vi "Read_AVI_to_Array.vi"(8 "Error in (no error)":errorcluster, 11 "AVI Path":path) -> (0 "Error out":errorcluster, 2 "Data Array":string[](array[string]), 3 "Image Array":T1[](array[plugin-control]))   [LabVIEW 2012]
doc: "This example shows how to read and write both image information and data to an AVI file. The example also shows how to read a specific frame in an AVI file. The VI opens an existing AVI file, adds time stamp information, sample waveform data, and writes a sample image and the data to a new AVI file. You then can read the image and data associated with a specific frame. Use the Flatten To String and Unflatten From String functions to write and read data in AVI files."
uses:
  <vilib>/vision/Image Controls.llb/IMAQ Image.ctl
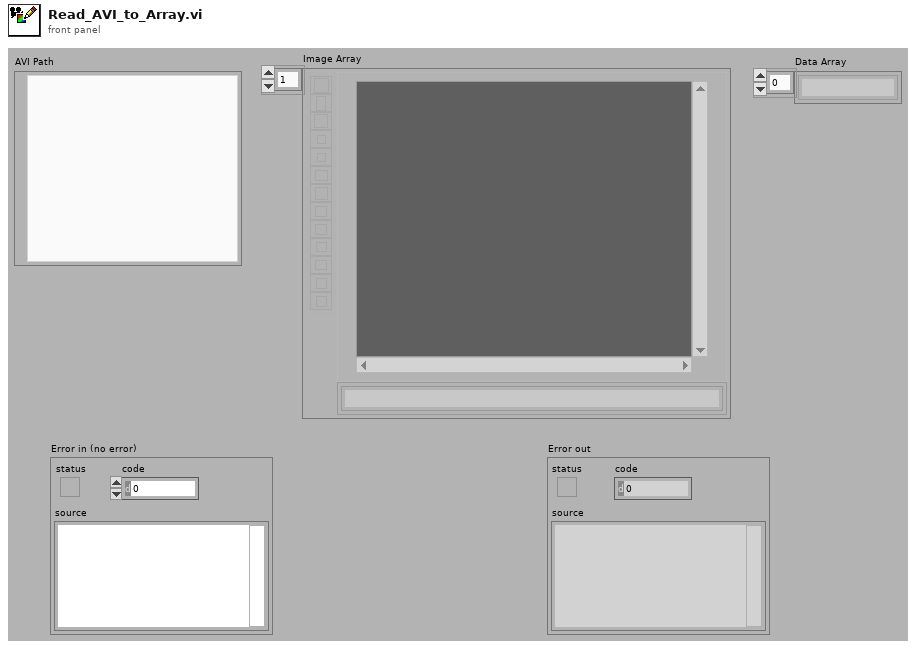
[diagram p1: front panel]
types:
  T1 = typedef "IMAQ Image.ctl" = refnum<image>
  T2 = typedef "Image Type" = u32
  T3 = typedef "AviRefnum.ctl" = refnum<k1>
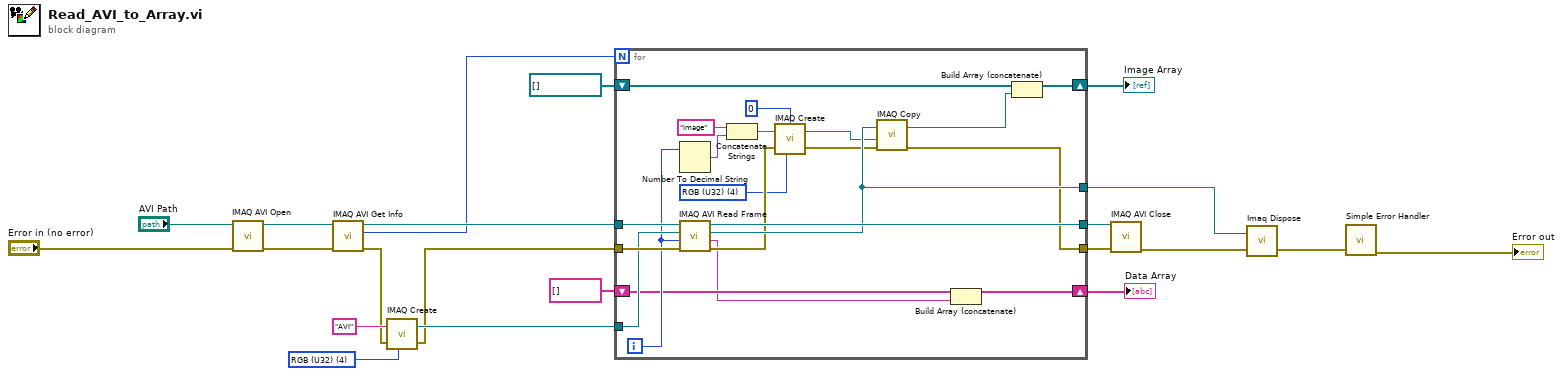
[diagram p0: block diagram]
diagram:
  w10 = T2 4 items=["Grayscale (U8)", "Grayscale (I16)", "Grayscale (SGL)", "Complex (CSG)", "RGB (U32)", "HSL (U32)", "RGB (U64)", "Grayscale (U16)"] ("Image Type")
  n1 = call "IMAQ AVI Open"("error in (no error)"="Error in (no error)", "AVI Path"="AVI Path") -> ("error out"=w14:errorcluster, "Avi Refnum"=w13:T3)  [unwired: 8 out]
  n2 = call "IMAQ AVI Get Info"("error in (no error)"=w14, "Avi Refnum"=w13) -> ("error out"=w8:errorcluster, "Number of Frames"=w9:u32, "Avi Refnum (duplicate)"=w12:T3)  [unwired: 5 in, 2 out]
  n3 = call "IMAQ Create"("Image Name"="AVI", "Image Type"=w10, "error in (no error)"=w8) -> ("New Image"=w19:T1, "error out"=w6:errorcluster)  [unwired: 1 in, 1 out]
  n4 = for {
    N: w9 -> [_]
    tunnel: [w38] -> w17
    tunnel: w19 -> [w39]
    tunnel: [w22] -> w16
    tunnel: [w40] -> w18
    tunnel: w12 -> [w42]
    tunnel: w6 -> [w41]
    shift-right: [w36] -> w1
    shift-left: T1[] [] ("Image Array") -> [w37]
    shift-right: [w25] -> w2
    shift-left: string[] [] ("Data Array") -> [w26]
    i -> [w27]
    w28 = T2 4 items=["Grayscale (U8)", "Grayscale (I16)", "Grayscale (SGL)", "Complex (CSG)", "RGB (U32)", "HSL (U32)", "RGB (U64)", "Grayscale (U16)"] ("Image Type")
    n5 = Number To Decimal String(number=w27) -> (decimal integer string=w33:string)  [unwired: 1 in]
    n6 = call "IMAQ AVI Read Frame"("error in (no error)"=w41, "Frame Number"=w27, "Image"=w39, "Avi Refnum"=w42) -> ("error out"=w30:errorcluster, "Data Out"=w24:string, "Image Out"=w38:T1, "Avi Refnum (duplicate)"=w40:T3)  [unwired: 1 in, 3 out]
    n7 = Concatenate Strings("image" ("string"), w33) -> (w35:string)
    n8 = call "IMAQ Create"("Border Size"=0, "Image Name"=w35, "Image Type"=w28, "error in (no error)"=w30) -> ("New Image"=w31:T1, "error out"=w29:errorcluster)  [unwired: 1 in]
    n9 = call "IMAQ Copy"("error in (no error)"=w29, "Image Dst"=w31, "Image Src"=w38) -> ("error out"=w22:errorcluster, "Image Dst Out"=w23:T1)  [unwired: 3 in]
    n10 = Build Array (concatenate)(w26, w24) -> (w25:string[])
    n11 = Build Array (concatenate)(w37, w23) -> (w36:T1[])
  }
  "Image Array" <- w1
  "Data Array" <- w2
  n12 = call "IMAQ AVI Close"("error in (no error)"=w16, "Avi Refnum"=w18) -> ("error out"=w15:errorcluster)  [unwired: 9 out]
  n13 = call "Imaq Dispose"("Image"=w17, "error in (no error)"=w15) -> ("error out"=w21:errorcluster)  [unwired: 1 in, 3 out]
  n14 = call <vilib>:"Simple Error Handler.vi"("error in (no error)"=w21) -> ("error out"=→"Error out":errorcluster)  [unwired: 1 in, 7 out]
